vi "Index ByteArray.vi"(4 "Size(s)":i32[](array[numeric]), 6 "Data Type":T1, 8 "error in (no error)":errorcluster, 10 "index":i32[](array[numeric]), 11 "values":u8[](array[numeric])) -> (0 "error out":errorcluster, 3 "values (indexed)":u8[](array[numeric]))   [LabVIEW 2021, in "Ring Buffer Strict Accessor.lvlib"]
uses:
  Ring Buffer Strict Accessor.lvlib
  DataType.ctl
  <vilib>/Utility/error.llb/Error Cluster From Error Code.vi
  <vilib>/ErrorRing/Error Ring.xnode
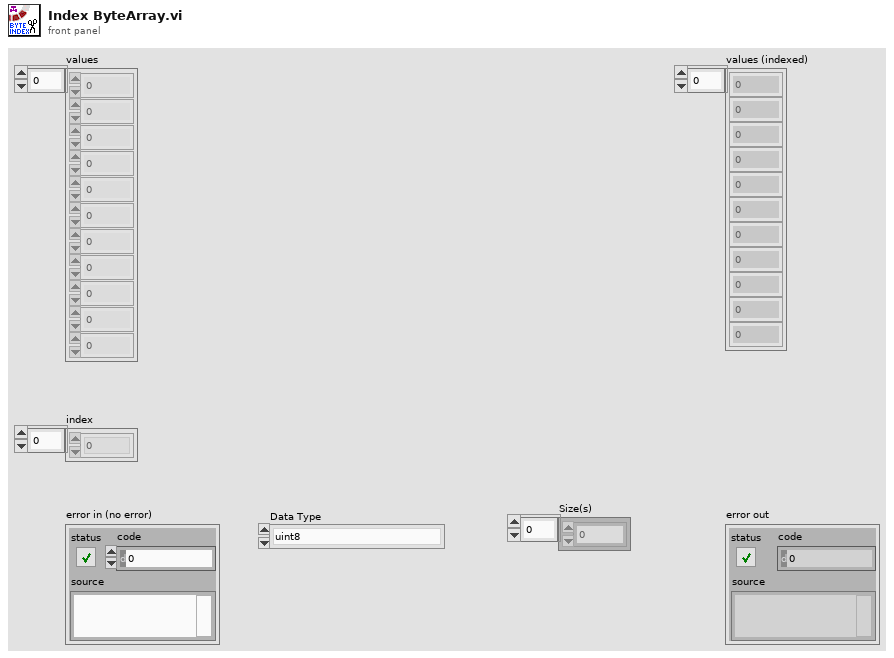
[diagram p1: front panel]
types:
  T1 = typedef "Ring Buffer Strict Accessor.lvlib/DataType.ctl" = enum16{"uint8", "uint16", "uint32", "uint64", "int8", "int16", "int32", "int64", "float", "double", "extended"}
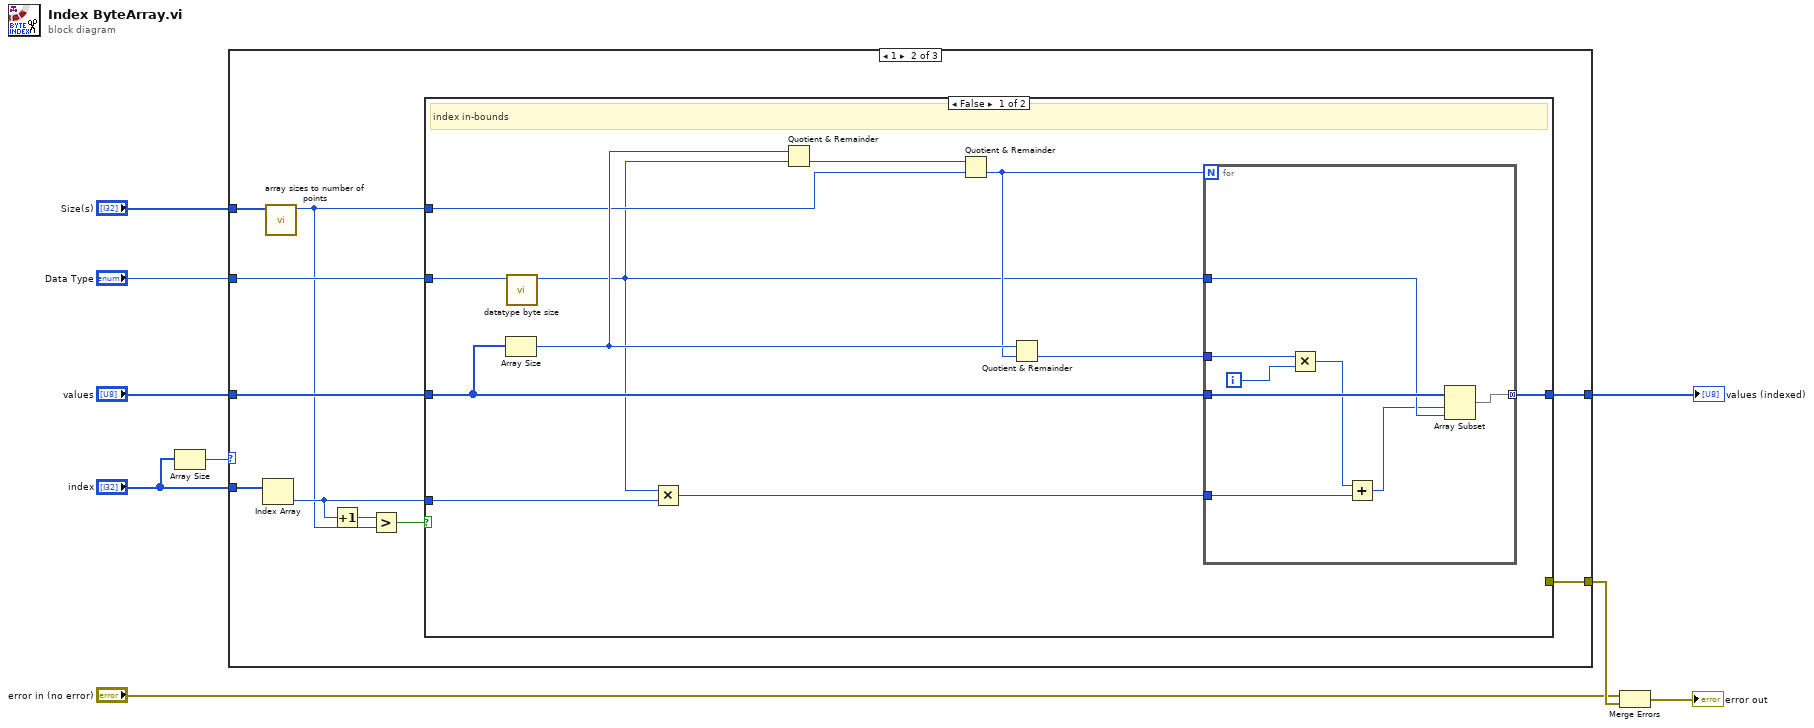
[diagram p0: block diagram]
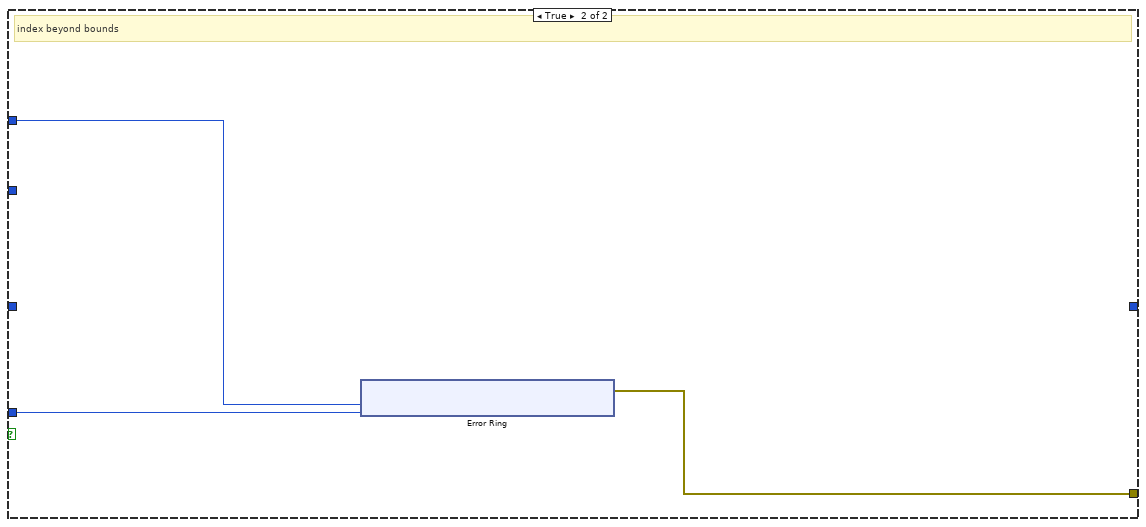
[diagram p3: hidden frame]
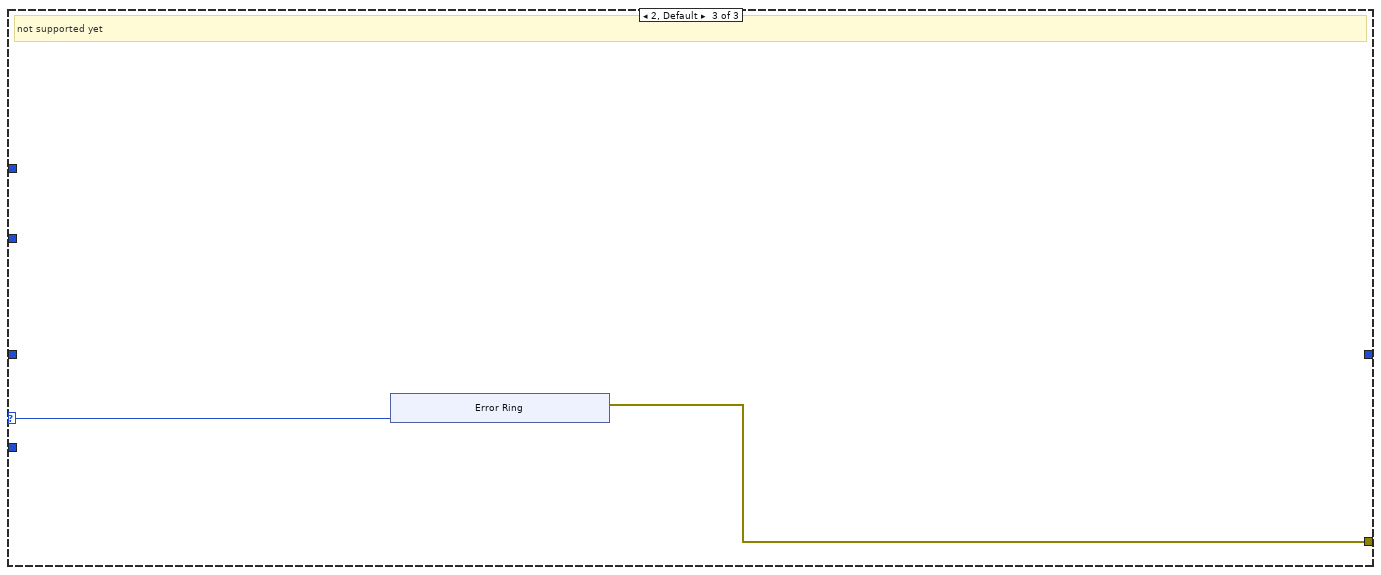
[diagram p4: hidden frame]
diagram:
  n1 = Array Size(array="index") -> (size(s)=w5:i32)
  n2 = case shown="1" w5 {
    selector: w5 -> [_ _ w52]
    tunnel: [w10 w20 _] -> w9
    tunnel: "index" -> [_ w17 _]
    tunnel: "Data Type" -> [_ w19 _]
    tunnel: "values" -> [w10 w18 _]
    tunnel: [_ w14 w51] -> w4
    tunnel: "Size(s)" -> [_ w12 _]
    frame 0 {
    }
    frame 1 {
      n3 = Index Array(array=w17) -> (element=w13:i32)  [unwired: 1 in]
      n4 = call "array sizes to number of points.vi"("Size(s)"=w12) -> ("#scalar values"=w11:i32)  [unwired: 10 in]
      n5 = Increment(x=w13) -> (x+1=w15:i32)
      n6 = Greater?(x=w15, y=w11) -> (0:w16:bool)
      n7 = case shown="False" w16 {
        tunnel: [w30 _] -> w20
        tunnel: w19 -> [w22 _]
        tunnel: w18 -> [w25 _]
        tunnel: w13 -> [w24 w41]
        tunnel: w11 -> [w23 w42]
        tunnel: [_ w40] -> w14
        frame False {
          # "index in-bounds"
          n8 = Array Size(array=w25) -> (size(s)=w29:i32)
          n9 = call "datatype byte size.vi"("Data Type"=w22) -> ("#bytes per scalar value"=w21:i32)  [unwired: 10 in]
          n10 = Multiply(x=w21, y=w24) -> (x*y=w26:i32)
          n11 = Quotient & Remainder(x=w29, y=w21) -> (floor(x/y)=w31:i32)  [unwired: 1 out]
          n12 = Quotient & Remainder(x=w31, y=w23) -> (floor(x/y)=w28:i32)  [unwired: 1 out]
          n13 = Quotient & Remainder(x=w29, y=w28) -> (floor(x/y)=w27:i32)  [unwired: 1 out]
          n14 = for {
            N: w28 -> [_]
            tunnel: w25 -> [w39]
            tunnel: [w38] -> w30 mode=concatenating
            tunnel: w21 -> [w37]
            tunnel: w27 -> [w36]
            tunnel: w26 -> [w33]
            i -> [w35]
            n15 = Multiply(x=w36, y=w35) -> (x*y=w34:i32)
            n16 = Add(x=w34, y=w33) -> (x+y=w32:i32)
            n17 = Array Subset(array=w39, index=w32, length=w37) -> (w38:u8[])
          }
        }
        frame True {
          # "index beyond bounds"
          n18 = xnode "Error Ring"("parameter 0"=w42, "parameter 1"=w41) -> ("error out"=w40:errorcluster)
        }
      }
    }
    frame 2, Default {
      # "not supported yet"
      n19 = xnode "Error Ring"("parameter 0"=w52) -> ("error out"=w51:errorcluster)
    }
  }
  "values (indexed)" <- w9
  n20 = Merge Errors("error in (no error)", w4) -> (→"error out":errorcluster)
